vi "Matrix_WithinTolerance.vi"(9 "Tolerance":dbl=1e-08, 10 "Matrix B":T1, 11 "Matrix A":T1) -> (0 "Error":bool, 3 "WithinTolerance":bool)   [LabVIEW 2019, in "Trajectory_Library.lvlib"]
uses:
  <vilib>/Analysis/Matrix/Datatypes/RealMatrix.ctl
  Trajectory_Library.lvlib
  <vilib>/Analysis/Matrix/NI_Matrix.lvlib
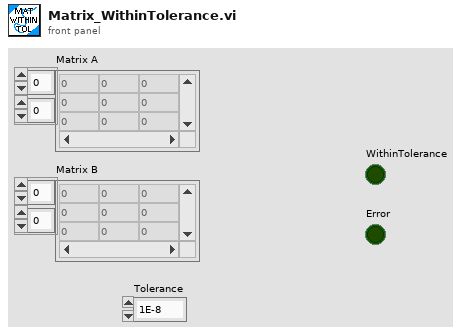
[diagram p1: front panel]
types:
  T1 = typedef "NI_Matrix.lvlib/RealMatrix.ctl" = dbl[][]
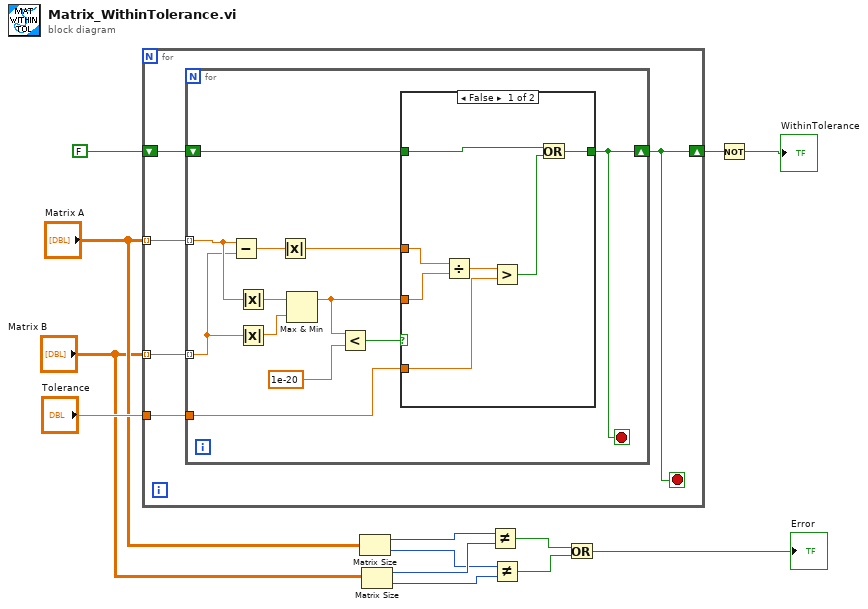
[diagram p0: block diagram]
diagram:
  n1 = for {
    tunnel: "Matrix A" -> [w17] mode=indexing
    tunnel: "Matrix B" -> [w18] mode=indexing
    shift-right: [w14] -> w11
    shift-left: FALSE -> [w16]
    tunnel: "Tolerance" -> [w15]
    stop <- w14 stop-if-true
    n2 = for {
      tunnel: w18 -> [w27] mode=indexing
      tunnel: w17 -> [w28] mode=indexing
      shift-right: [w19] -> w14
      shift-left: w16 -> [w23]
      tunnel: w15 -> [w20]
      stop <- w19 stop-if-true
      n3 = Subtract(x=w28, y=w27) -> (x-y=w30:dbl)
      n4 = Absolute Value(x=w28) -> (abs(x)=w26:dbl)
      n5 = Absolute Value(x=w27) -> (abs(x)=w25:dbl)
      n6 = Absolute Value(x=w30) -> (abs(x)=w22:dbl)
      n7 = Max & Min(x=w26, y=w25) -> (max(x,y)=w21:dbl)  [unwired: 1 out]
      n8 = Less?(x=w21, y=1e-20) -> (x < y?=w24:bool)
      n9 = case shown="False" w24 {
        tunnel: w23 -> [w31 w38]
        tunnel: [w33 w38] -> w19
        tunnel: w22 -> [w37 _]
        tunnel: w21 -> [w36 _]
        tunnel: w20 -> [w34 _]
        frame False {
          n10 = Divide(x=w37, y=w36) -> (x/y=w35:dbl)
          n11 = Greater?(x=w35, y=w34) -> (0:w32:bool)
          n12 = Or(x=w31, y=w32) -> (x .or. y?=w33:bool)
        }
        frame True {
        }
      }
    }
  }
  n13 = Matrix Size(0:"Matrix A") -> (1:w7:i32, 2:w5:i32)
  n14 = Matrix Size(0:"Matrix B") -> (1:w6:i32, 2:w4:i32)
  n15 = Not Equal?(x=w7, y=w6) -> (x != y?=w3:bool)
  n16 = Not Equal?(x=w5, y=w4) -> (x != y?=w2:bool)
  n17 = Or(x=w3, y=w2) -> (x .or. y?=→"Error":bool)
  n18 = Not(x=w11) -> (.not. x?=→"WithinTolerance":bool)
